vi "DT_Triangle Manager_Default Ghost Index.vi"() -> (3 "ghost index":i32)   [LabVIEW 2020, in "NI_AAL_Geometry.lvlib"]
uses:
  <vilib>/Analysis/NI_AAL_Geometry.lvlib
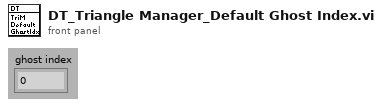
[diagram p1: front panel]
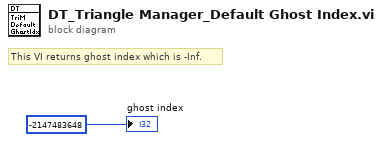
[diagram p0: block diagram]
diagram:
  # "This VI returns ghost index which is -Inf."
  "ghost index" <- -2147483648 ("element")
